vi "ROI entry screen-Extract userROI Motor Z plane.vi"(11 "ROI management Input cluster":T1) -> (3 "Motor Z plane":dbl)   [LabVIEW 2017]
uses:
  Typedefs/ROI management Input cluster.ctl
  Typedefs/ROI ID Enum.ctl
panel:
  # "X Start\nY Start\nX Stop\nY Stop"
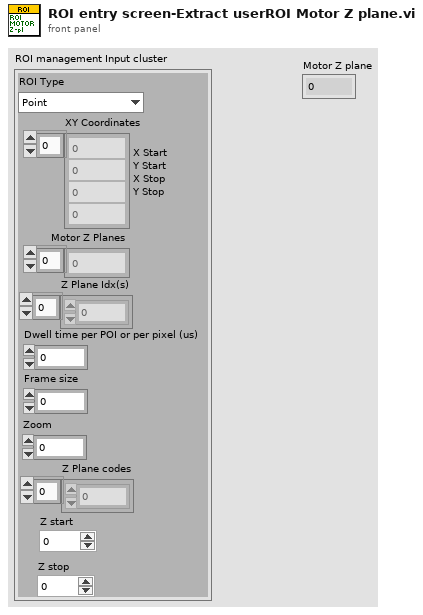
[diagram p1: front panel]
types:
  T1 = typedef "ROI management Input cluster.ctl" = cluster{"ROI Type":T2, "XY Coordinates":i32[], "Motor Z Planes":dbl[], "Dwell time per POI or per pixel (us)":dbl, "Frame size":i32, "Zoom":dbl, "Z Plane Idx(s)":i32[], "Z Plane codes":u8[], "Z start":dbl, "Z stop":dbl}
  T2 = typedef "ROI ID Enum.ctl" = enum16{"Point", "MiniScan", "Comp. MiniScan", "Rectangle", "Comp. volume", "Arb. plane point", "None"}
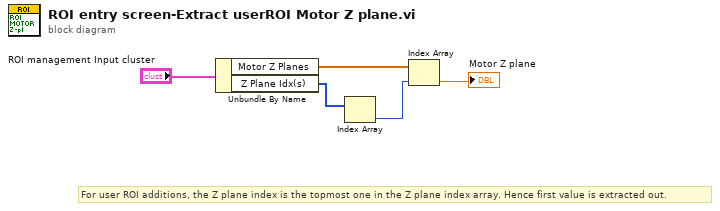
[diagram p0: block diagram]
diagram:
  # "For user ROI additions, the Z plane index is the topmost one in the Z plane index array. Hence first value is extracted out."
  n1 = Unbundle By Name("ROI management Input cluster") -> ("Motor Z Planes"=w2:dbl[], "Z Plane Idx(s)"=w4:i32[])
  n2 = Index Array(array=w4) -> (element=w3:i32)  [unwired: 1 in]
  n3 = Index Array(array=w2, index=w3) -> (element=→"Motor Z plane":dbl)
